vi "Write testActiveIsTrue.vi"(10 "testActiveIsTrue":bool, 11 "TestMonitor in":refnum<class "TestMonitor.lvclass">) -> (3 "TestMonitor out":refnum<class "TestMonitor.lvclass">)   [LabVIEW 2013, in "TestMonitor.lvclass"]
uses:
  TestMonitor.lvclass
  TestMonitor.lvclass/TestMonitor.ctl
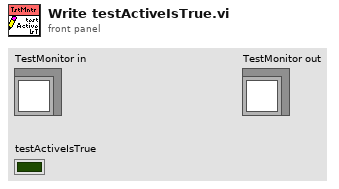
[diagram p1: front panel]
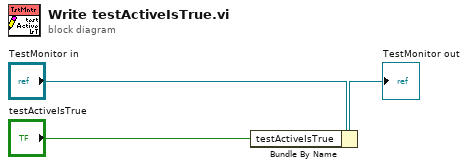
[diagram p0: block diagram]
diagram:
  n1 = Bundle By Name(cluster="TestMonitor in", "testActiveIsTrue"="testActiveIsTrue") -> (→"TestMonitor out":refnum<class "TestMonitor.lvclass">)
